vi "CalculateRandG.vi"(8 "V2":i32, 9 "V1":i32, 10 "Current":i32, 11 "Lockin[ ]":dbl[](array[numeric])) -> (2 "G(Siements)":dbl, 3 "R(ohms)":dbl)   [LabVIEW 2016, in "Transport.lvclass"]
uses:
  Transport.lvclass
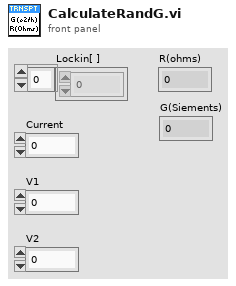
[diagram p1: front panel]
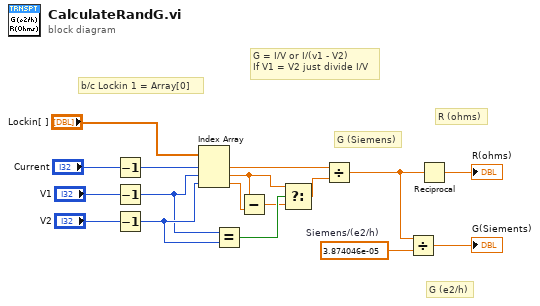
[diagram p0: block diagram]
diagram:
  w6 = 3.874046e-05  # Siemens/(e2/h)
  # "G (e2/h)"
  # "R (ohms)"
  # "G (Siemens)"
  # "b/c Lockin 1 = Array[0]"
  # "G = I/V or I/(v1 - V2)\nIf V1 = V2 just divide I/V"
  n1 = Decrement(x="Current") -> (x-1=w7:i32)
  n2 = Decrement(x="V1") -> (x-1=w11:i32)
  n3 = Decrement(x="V2") -> (x-1=w12:i32)
  n4 = Index Array(array="Lockin[ ]", index #1=w7, index #2=w11, index #3=w12) -> (element #1=w5:dbl, element #2=w10:dbl, element #3=w8:dbl)
  n5 = Equal?(x=w11, y=w12) -> (x = y?=w13:bool)
  n6 = Subtract(x=w10, y=w8) -> (x-y=w9:dbl)
  n7 = Select(t=w10, s=w13, f=w9) -> (s? t:f=w4:dbl)
  n8 = Divide(x=w5, y=w4) -> (x/y=w2:dbl)
  n9 = Divide(x=w2, y=w6) -> (x/y=→"G(Siements)":dbl)
  n10 = Reciprocal(x=w2) -> (1/x=→"R(ohms)":dbl)
